vi "Read.vi"(8 "error in (no error)":errorcluster, 11 "Double Float.lvclass in":refnum<class "Divide_INT.lvclass">) -> (0 "error out":errorcluster, 2 "Value":T1, 3 "Double Float.lvclass out":refnum<class "Divide_INT.lvclass">)   [LabVIEW 2021, in "Divide_INT.lvclass"]
uses:
  Divide_INT.lvclass
  Abs_Types/Double Float/Support/Type.ctl
  Divide_INT.lvclass/Divide_INT.ctl
  Abs_Types/Integer/Abs_Integer.lvclass
  Abs_Types/Numeric/Abs_Numeric.lvclass
  Abs_Types/Double Float/Abs_Double Float.lvclass
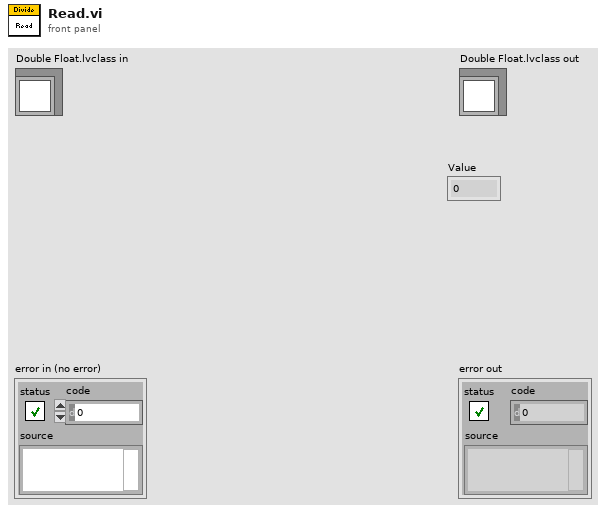
[diagram p1: front panel]
types:
  T1 = typedef "Abs_Double Float.lvclass/Type.ctl" = dbl
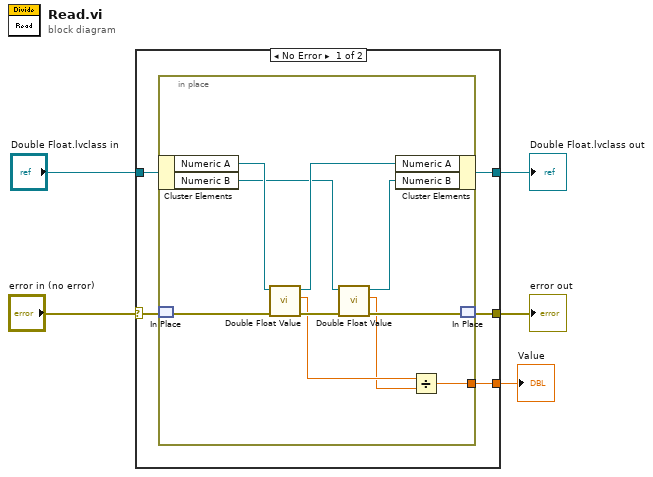
[diagram p0: block diagram]
diagram:
  n1 = case shown="No Error" "error in (no error)" {
    selector: "error in (no error)" -> [w9 w21]
    tunnel: "Double Float.lvclass in" -> [w10 w22]
    tunnel: [w8 w22] -> w3
    tunnel: [w7 w21] -> w2
    tunnel: [w6 _] -> w1
    frame No Error {
      n2 = in-place {
        in-place-border: [w11] -> w6
        n3 = in-place-cluster #1(w10) -> ("Numeric A"=w20:refnum<class "Abs_Integer.lvclass">, "Numeric B"=w17:refnum<class "Abs_Numeric.lvclass">)
        n4 = in-place-match #2(w9) -> (w18:errorcluster)
        n5 = call-dynamic "Double Float Value.vi"("error in (no error)"=w18, "Numeric in"=w20) -> ("error out"=w15:errorcluster, "Double"=w13:dbl, "Numeric out"=w19:refnum<class "Abs_Integer.lvclass">)  [unwired: 7 in]
        n6 = call-dynamic "Double Float Value.vi"("error in (no error)"=w15, "Numeric in"=w17) -> ("error out"=w14:errorcluster, "Double"=w12:dbl, "Numeric out"=w16:refnum<class "Abs_Numeric.lvclass">)  [unwired: 7 in]
        n7 = in-place-cluster #1("Numeric A"=w19, "Numeric B"=w16) -> (w8:refnum<class "Divide_INT.lvclass">)
        n8 = Divide(x=w13, y=w12) -> (x/y=w11:dbl)
        n9 = in-place-match #2(w14) -> (w7:errorcluster)
      }
    }
    frame Error {
    }
  }
  "error out" <- w2
  "Double Float.lvclass out" <- w3
  "Value" <- w1
